vi "decrypt data from file.vi"() -> ()   [LabVIEW 2025]
panel:
  out "Array":string[](array[string])
  out "Output":string
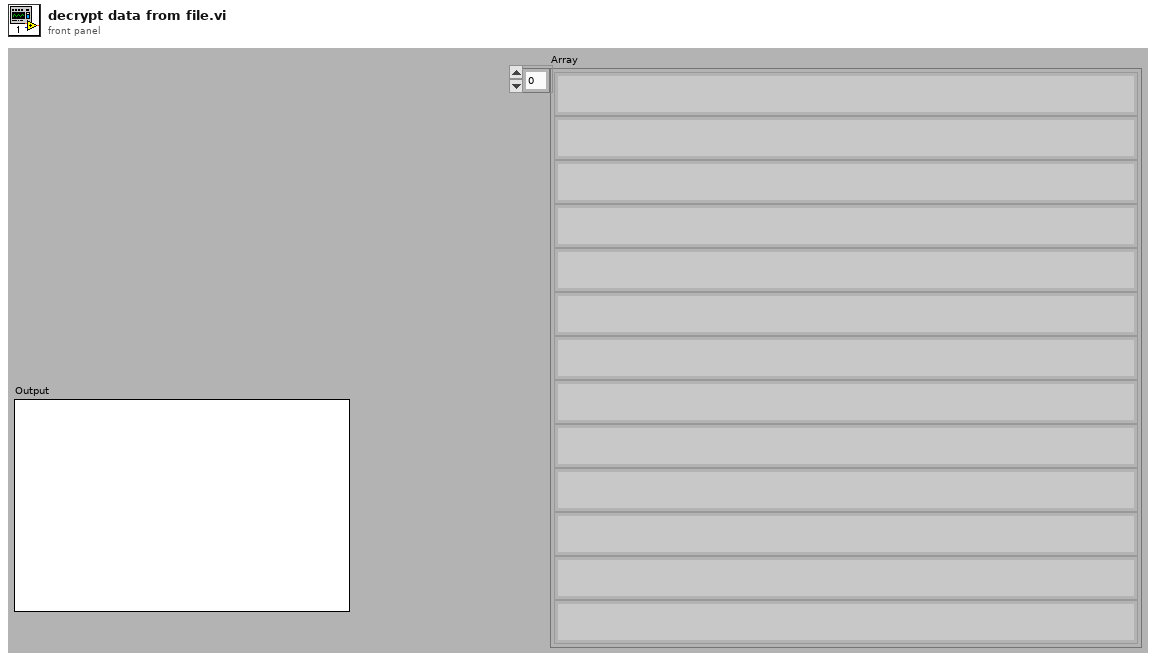
[diagram p1: front panel]
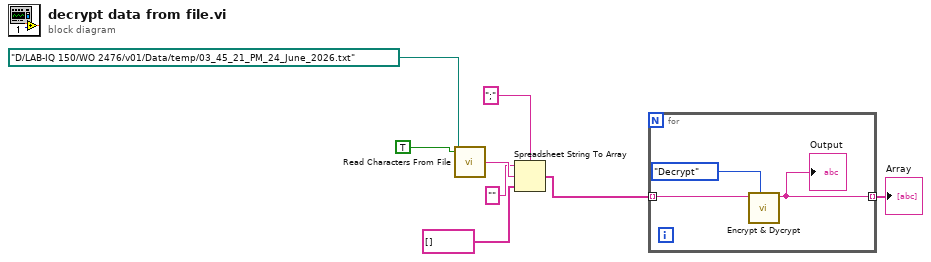
[diagram p0: block diagram]
diagram:
  n1 = call <vilib>:"Read Characters From File.vi"("file path (dialog if empty)"=path "D:/LAB-IQ 150/WO 2476/v01/Data/temp/03_45_21_PM_24_June_2026.txt", "convert eol? (no:F)"=TRUE ("append to file? (new file:F)")) -> ("character string"=w6:string)  [unwired: 4 in, 3 out]
  n2 = Spreadsheet String To Array(delimiter (Tab)=";" ("string"), format string="", spreadsheet string=w6, array type (2D Dbl)=string[] []) -> (array=w4:string[])
  n3 = for {
    tunnel: w4 -> [w10] mode=indexing
    tunnel: [w9] -> w3 mode=indexing
    n4 = call "Encrypt & Dycrypt.vi"("Enum"=enum16{"Encrypt", "Decrypt"}."Decrypt", "Input"=w10) -> ("Output"=w9:string)  [unwired: 8 in, 1 out]
    "Output" <- w9
  }
  "Array" <- w3
